vi "CRYStep Contents Init.vi"() -> ()   [LabVIEW 2013]
uses:
  CRYMainGlobal.vi
  CRYProject/CRYProject Editor Global.vi
panel:
  out "status":bool
  # "Loading Step Files in Add Step Global Variables."
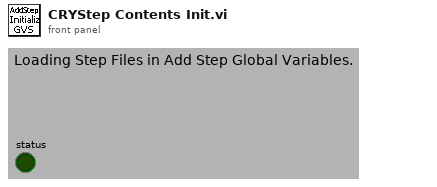
[diagram p1: front panel]
types:
  T1 = cluster{"Content":string, "Name":string, "Level":u32, "Category":string}[]
  T2 = cluster{"Content":string, "Name":string, "Level":u32, "Category":string}
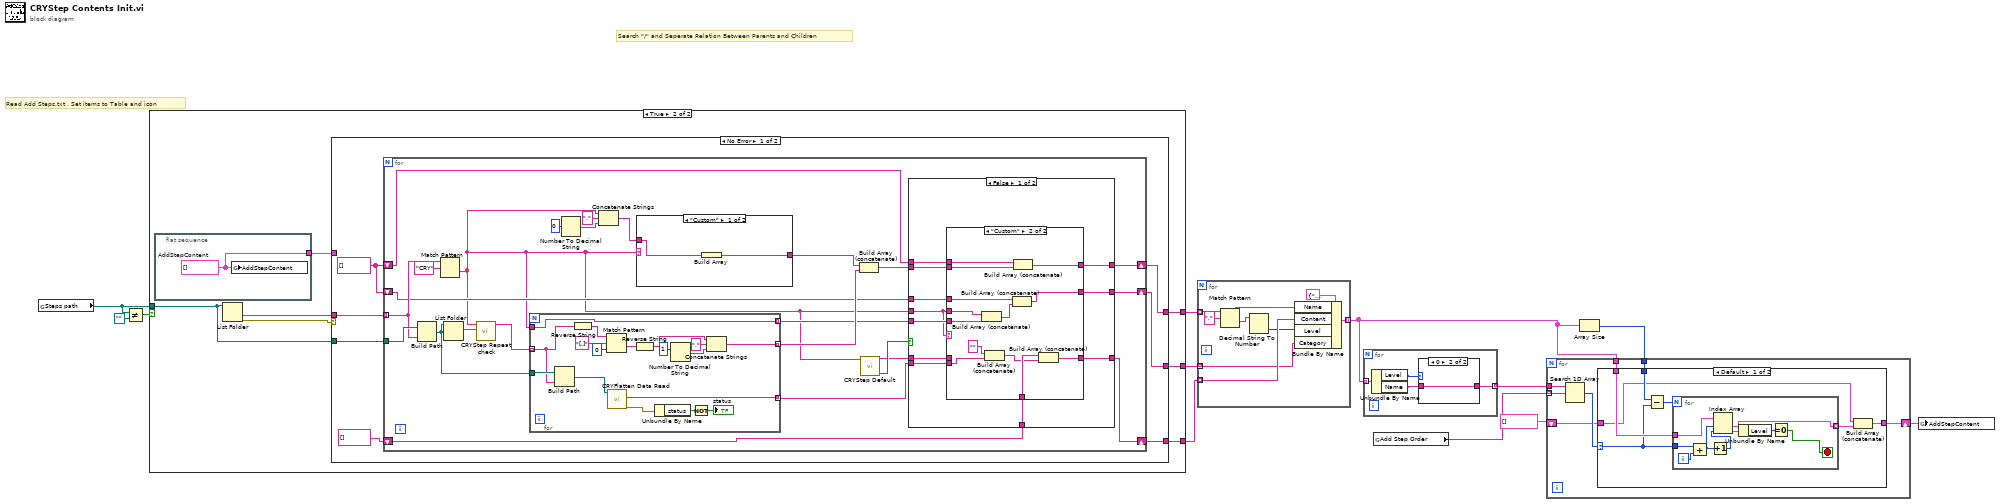
[diagram p0: block diagram]
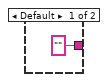
[diagram p3: hidden frame]
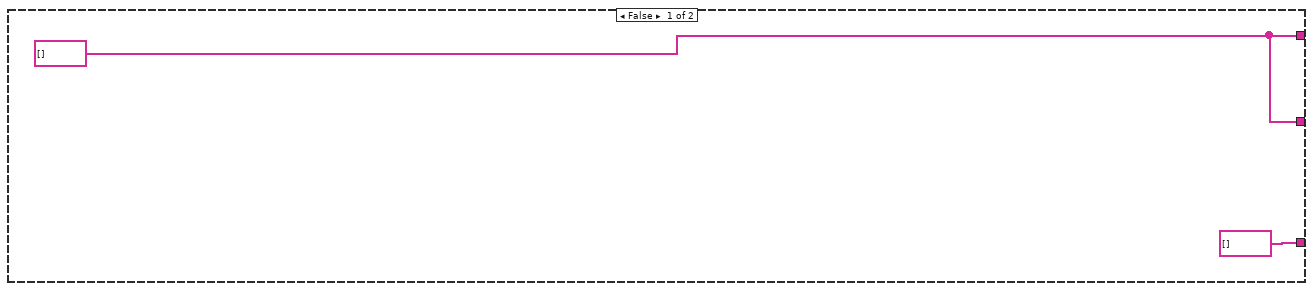
[diagram p4: hidden frame]
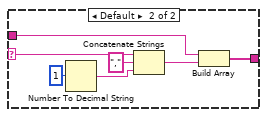
[diagram p5: hidden frame]
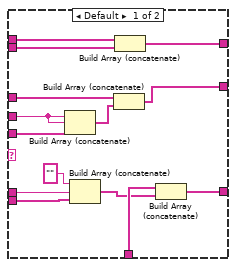
[diagram p6: hidden frame]
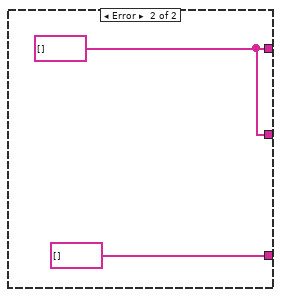
[diagram p8: hidden frame]
diagram:
  # "Search \"/\" and Seperate Relation Between Parents and Children"
  # "Read Add Steps.txt , Set items to Table and icon"
  n1 = global read "CRYMainGlobal.vi" "Steps path"() -> (w4:path)
  n2 = Not Equal?(x=w4, y=path "") -> (x != y?=w12:bool)
  n3 = case shown="True" w12 {
    tunnel: w4 -> [_ w21]
    tunnel: [w13 w20] -> w9
    tunnel: [string[] [] ("appended array") w19] -> w10
    tunnel: [w13 w15] -> w1
    frame False {
      w13 = string[] []
    }
    frame True {
      n4 = flat-sequence {
        tunnel: [w22] -> w16
        frame #0 {
          w22 = T1 []  # AddStepContent
          n5 = global write "CRYProject Editor Global.vi" "AddStepContent"(w22) -> ()
        }
      }
      n6 = List Folder(path=w21) -> (folder names=w18:string[], error out=w17:errorcluster)  [unwired: 1 in, 4 out]
      n7 = case shown="No Error" w17 {
        tunnel: w21 -> [w29 _]
        tunnel: [w28 w121] -> w20
        tunnel: [w26 string[] [] ("appended array")] -> w19
        tunnel: w18 -> [w25 _]
        tunnel: w16 -> [_ _]
        tunnel: [w23 w121] -> w15
        frame No Error {
          w24 = string[] [] ("appended array")
          n8 = for {
            tunnel: w25 -> [w48] mode=indexing
            tunnel: w29 -> [w53]
            shift-right: [w38] -> w28
            shift-left: w24 -> [w37]
            shift-right: [w40] -> w26
            shift-left: string[] [] ("appended array") -> [w41]
            shift-right: [w33] -> w23
            shift-left: w24 -> [w32]
            n9 = Build Path(base path=w53, name or relative path=w48) -> (appended path=w47:path)
            n10 = Match Pattern(string=w48, regular expression="CRY" ("string")) -> (after substring=w30:string)  [unwired: 4 out]
            n11 = List Folder(path=w47) -> (filenames=w46:string[])  [unwired: 1 in, 5 out]
            n12 = call "CRYStep Repeat check.vi"("In String Array"=w46, "In String for Compare"=w30) -> ("Out String Array"=w45:string[])  [unwired: 9 out]
            n13 = for {
              tunnel: w45 -> [w109] mode=indexing
              tunnel: [w113] -> w39 mode=indexing
              tunnel: w30 -> [w104]
              tunnel: w47 -> [w117]
              tunnel: [w111] -> w42 mode=indexing
              tunnel: [w104] -> w31 mode=indexing
              n14 = Build Path(base path=w117, name or relative path=w109) -> (appended path=w105:path)
              n15 = Reverse String(1:w109) -> (0:w108:string)
              n16 = Match Pattern(string=w108, regular expression="[.]", offset (0)=0) -> (after substring=w107:string)  [unwired: 3 out]
              n17 = call "CRYFlatten Data Read.vi"("Path In"=w105) -> ("error out"=w110:errorcluster, "Flatten Data Out"=w111:string)  [unwired: 6 in, 1 out]
              n18 = Reverse String(1:w107) -> (0:w106:string)
              n19 = Unbundle By Name(w110) -> ("status"=w116:bool)
              n20 = Number To Decimal String(number=1) -> (decimal integer string=w120:string)  [unwired: 1 out]
              n21 = Not(x=w116) -> (.not. x?=→"status":bool)
              n22 = Concatenate Strings(w106, "," ("string"), w120) -> (w113:string)
            }
            n23 = Number To Decimal String(number=0) -> (decimal integer string=w50:string)  [unwired: 1 out]
            n24 = Concatenate Strings(w30, "," ("string"), w50) -> (w34:string)
            n25 = case shown="\"Custom\"" w30 {
              selector: w30 -> [_ w56]
              tunnel: [w54 w58] -> w35
              tunnel: w34 -> [w55 w57]
              frame "Custom" {
                n26 = Build Array(w55) -> (w54:string[])
              }
              frame Default {
                n27 = Number To Decimal String(number=1) -> (decimal integer string=w62:string)  [unwired: 1 out]
                n28 = Concatenate Strings(w56, "," ("string"), w62) -> (w59:string)
                n29 = Build Array(w57, w59) -> (w58:string[])
              }
            }
            n30 = Build Array (concatenate)(w35, w39) -> (w36:string[])
            n31 = call "CRYStep Default.vi"("Category Name"=w30) -> ("status"=w44:bool, "Flatten Step"=w43:string)  [unwired: 9 out]
            n32 = case shown="False" w44 {
              tunnel: w43 -> [w73 _]
              tunnel: w42 -> [w72 _]
              tunnel: w41 -> [w71 w103]
              tunnel: [w70 w103] -> w40
              tunnel: w37 -> [w69 w102]
              tunnel: [w68 w102] -> w38
              tunnel: w36 -> [w67 _]
              tunnel: [w64 w101] -> w33
              tunnel: w32 -> [w65 w101]
              tunnel: w31 -> [w66 _]
              tunnel: w30 -> [w63 _]
              frame False {
                n33 = case shown="\"Custom\"" w63 {
                  tunnel: w73 -> [w86 _]
                  tunnel: w72 -> [w85 w88]
                  tunnel: w71 -> [w84 w99]
                  tunnel: [w82 w97] -> w70
                  tunnel: w69 -> [w81 w96]
                  tunnel: [w80 w95] -> w68
                  tunnel: w67 -> [w79 w94]
                  tunnel: w66 -> [w78 w93]
                  tunnel: w63 -> [w77 w92]
                  tunnel: w65 -> [w76 w91]
                  tunnel: [w74 w89] -> w64
                  frame Default {
                    n34 = Build Array (concatenate)(w77, w77, w78) -> (w75:string[])
                    n35 = Build Array (concatenate)("" ("element"), w86, w85) -> (w83:string[])
                    n36 = Build Array (concatenate)(w76, w75) -> (w74:string[])
                    n37 = Build Array (concatenate)(w81, w79) -> (w80:string[])
                    n38 = Build Array (concatenate)(w84, w83) -> (w82:string[])
                  }
                  frame "Custom" {
                    n39 = Build Array (concatenate)(w92, w93) -> (w90:string[])
                    n40 = Build Array (concatenate)("" ("element"), w88) -> (w98:string[])
                    n41 = Build Array (concatenate)(w91, w90) -> (w89:string[])
                    n42 = Build Array (concatenate)(w96, w94) -> (w95:string[])
                    n43 = Build Array (concatenate)(w99, w98) -> (w97:string[])
                  }
                }
              }
              frame True {
              }
            }
          }
        }
        frame Error {
          w121 = string[] [] ("appended array")
        }
      }
    }
  }
  n44 = for {
    tunnel: w9 -> [w130] mode=indexing
    tunnel: w10 -> [w128] mode=indexing
    tunnel: [w125] -> w7 mode=indexing
    tunnel: w1 -> [w123] mode=indexing
    n45 = Match Pattern(string=w130, regular expression=",") -> (before substring=w127:string, after substring=w129:string)  [unwired: 3 out]
    n46 = Decimal String To Number(string=w129) -> (number=w126:i32)  [unwired: 3 out]
    n47 = Bundle By Name(cluster=T2 {"Content"="", "Name"="", "Level"=0, "Category"=""}, "Name"=w127, "Content"=w128, "Level"=w126, "Category"=w123) -> (w125:T2)
  }
  n48 = for {
    tunnel: w7 -> [w135] mode=indexing
    tunnel: [w132] -> w8 mode=indexing
    n49 = Unbundle By Name(w135) -> ("Level"=w134:u32, "Name"=w133:string)
    n50 = case shown="0" w134 {
      tunnel: ["" ("Name") w137] -> w132
      tunnel: w133 -> [_ w137]
      frame Default {
      }
      frame 0 {
      }
    }
  }
  n51 = global read "CRYMainGlobal.vi" "Add Step Order"() -> (w5:string[])
  n52 = Array Size(array=w7) -> (size(s)=w6:i32)
  n53 = for {
    tunnel: w5 -> [w143] mode=indexing
    tunnel: w8 -> [w144]
    tunnel: w7 -> [w141]
    tunnel: w6 -> [w140]
    shift-right: [w138] -> w2
    shift-left: T1 [] ("AddStepContent") -> [w139]
    n54 = Search 1D Array(1D array=w144, element=w143) -> (index of element=w142:i32)  [unwired: 1 in]
    n55 = case shown="Default" w142 {
      selector: w142 -> [w149 _]
      tunnel: w141 -> [w151 _]
      tunnel: w140 -> [w150 _]
      tunnel: [w146 w161] -> w138
      tunnel: w139 -> [w147 w161]
      frame Default {
        n56 = Subtract(x=w150, y=w149) -> (x-y=w148:i32)
        n57 = for {
          N: w148 -> [_]
          tunnel: w149 -> [w160]
          tunnel: w151 -> [w159]
          tunnel: [w153] -> w145 mode=indexing
          i -> [w158]
          stop <- w152 stop-if-true
          n58 = Add(x=w160, y=w158) -> (x+y=w157:i32)
          n59 = Increment(x=w157) -> (x+1=w156:i32)
          n60 = Index Array(array=w159, index #1=w157, index #2=w156) -> (element #1=w153:T2, element #2=w155:T2)
          n61 = Unbundle By Name(w155) -> ("Level"=w154:u32)
          n62 = Equal To 0?(x=w154) -> (x = 0?=w152:bool)
        }
        n63 = Build Array (concatenate)(w147, w145) -> (w146:T1)
      }
      frame -1 {
      }
    }
  }
  n64 = global write "CRYProject Editor Global.vi" "AddStepContent"(w2) -> ()
